vi "launcher.vi"   [LabVIEW 2023]
uses:
  <vilib>/ActorFramework/Actor/Actor.lvclass
  InterferometerUI.lvclass
  Applications/National Instruments/LabVIEW 2023 64-bit/vi.lib/ActorFramework/Actor/Actor.lvclass
  Users/alexandrosspiliotis/Documents/LV_DAQ_Project/InterferometryUI/InterferometrUI/InterferometrUI/InterferometerUI.lvclass
  Users/alexandrosspiliotis/Documents/LV_DAQ_Project/Cameras_LV/CameraDAQ/CameraDAQ.lvclass
  Users/alexandrosspiliotis/Documents/LV_DAQ_Project/Cameras_LV/InitDeinitComm/InitDeinitComm.lvclass
  Users/alexandrosspiliotis/Documents/LV_DAQ_Project/TranslationStage/TranslationStagesComm/TranslationStagesComm.lvclass
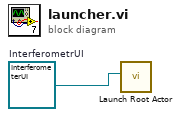
[diagram p0: block diagram]
diagram:
  w1 = refnum<class "InterferometerUI.lvclass"> refnum  # InterferometrUI
  n1 = call <vilib>:"Launch Root Actor.vi"("Actor"=w1) -> ()  [unwired: 9 in, 2 out]
